vi "set_edge_attribute.vi"(7 "attribute-name":string, 8 "error in (no error)":errorcluster, 9 "attribute-value":variant, 10 "edge":refnum<class "Edge.lvclass">, 11 "graph":refnum<class "Graph.lvclass">) -> (0 "error out":errorcluster, 3 "graph-out":refnum<class "Graph.lvclass">)   [LabVIEW 2020, in "graph.lvlib" / "Graph.lvclass"]
uses:
  Graph.lvclass
  Edge/Edge.lvclass
  Graph.lvclass/Graph.ctl
  <vilib>/Utility/miscctls.llb/LVMapReplaceAction.ctl
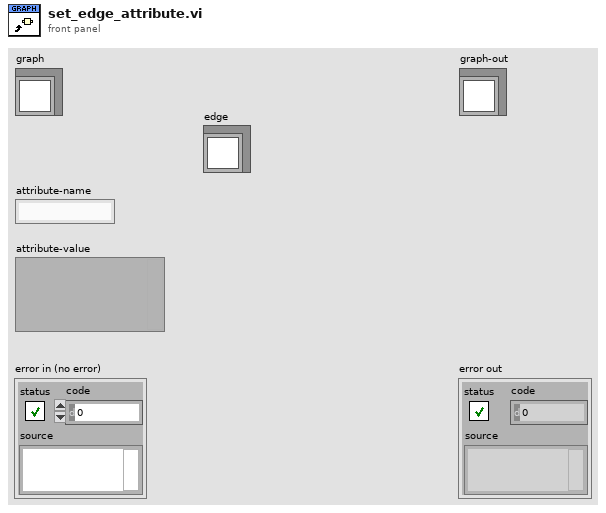
[diagram p1: front panel]
types:
  T1 = typedef "LVMapReplaceAction.ctl" = enum32{"Modify Entry only if found", "Add or Modify Entry", "Delete Entry"}
  T2 = typedef "graph.lvlib/Graph.lvclass/edge-definition-cluster.ctl" = cluster{"source-id":refnum<class "ID.lvclass">, "sink-id":refnum<class "ID.lvclass">}
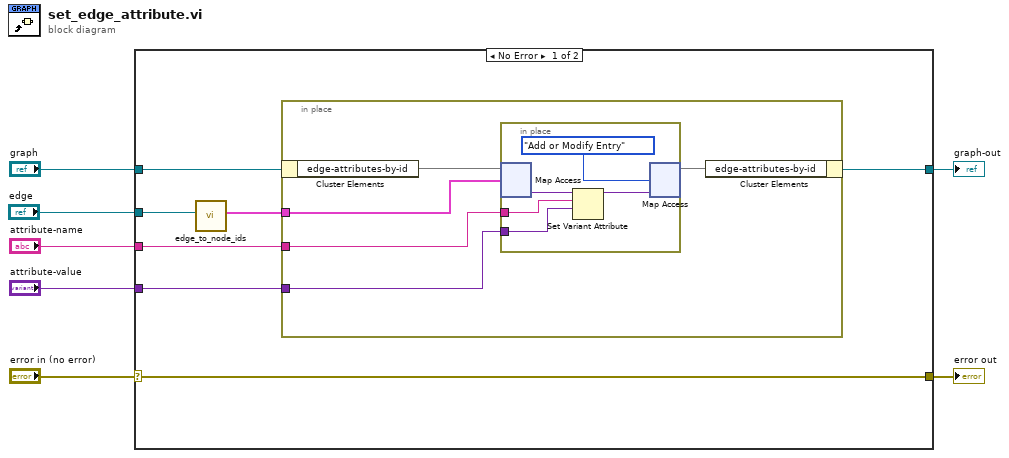
[diagram p0: block diagram]
diagram:
  n1 = case shown="No Error" "error in (no error)" {
    selector: "error in (no error)" -> [w14 w26]
    tunnel: [w14 w26] -> w6
    tunnel: [w11 w25] -> w4
    tunnel: "graph" -> [w10 w25]
    tunnel: "attribute-name" -> [w13 _]
    tunnel: "attribute-value" -> [w12 _]
    tunnel: "edge" -> [w8 _]
    frame No Error {
      n2 = call "edge_to_node_ids.vi"("edge"=w8) -> ("node-ids-cluster"=w9:T2)  [unwired: 10 in]
      n3 = in-place {
        in-place-border: w13 -> [w17]
        in-place-border: w12 -> [w16]
        in-place-border: w9 -> [w15]
        n4 = in-place-cluster #1(w10) -> ("edge-attributes-by-id"=w19:map{T2, variant})
        n5 = in-place {
          in-place-border: w17 -> [w22]
          in-place-border: w16 -> [w21]
          n6 = in-place-map #2(w19, w15) -> (w24:variant)  [unwired: 1 in, 1 out]
          n7 = Set Variant Attribute(Variant=w24, name=w22, value=w21) -> (Variant out=w23:variant)  [unwired: 1 in, 2 out]
          n8 = in-place-map #2(w23, LVMapReplaceAction."Add or Modify Entry" ("action")) -> (w18:map{T2, variant})  [unwired: 2 out]
        }
        n9 = in-place-cluster #1("edge-attributes-by-id"=w18) -> (w11:refnum<class "Graph.lvclass">)
      }
    }
    frame Error {
    }
  }
  "error out" <- w6
  "graph-out" <- w4
